vi "Initialize Daemon.vi"(8 "error in (no error)":errorcluster, 9 "data model":refnum<class "Device Data Model.lvclass">, 10 "transmission data unit":refnum<class "Transmission Data Unit.lvclass">, 11 "serial slave in":refnum<class "Serial Slave.lvclass">) -> (0 "error out":errorcluster, 3 "serial slave out":refnum<class "Serial Slave.lvclass">)   [LabVIEW 2018, in "SubVIs.lvlib" / "Serial Slave.lvclass"]
doc: "This provides an interface for the slave to launch a protocol daemon."
uses:
  Serial Slave.lvclass
  Transmission Data Unit.lvclass
  Device Data Model.lvclass
  Serial Data Unit.lvclass
  C:/OCC/ICM/Source Distributions/Buses/Transmission Data Unit.lvclass
  Serial Slave.lvclass/Serial Slave.ctl
  Transmission Data Unit.lvclass/Transmission Data Unit.ctl
  Read VISA resource name.vi
  Read Baud Rate.vi
  Read Parity.vi
  Read Flow Control.vi
  Network Slave.lvclass
  SubVIs.lvlib
  Serial Shared Components.lvlib
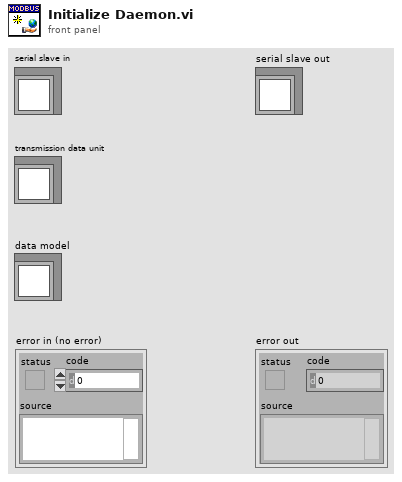
[diagram p1: front panel]
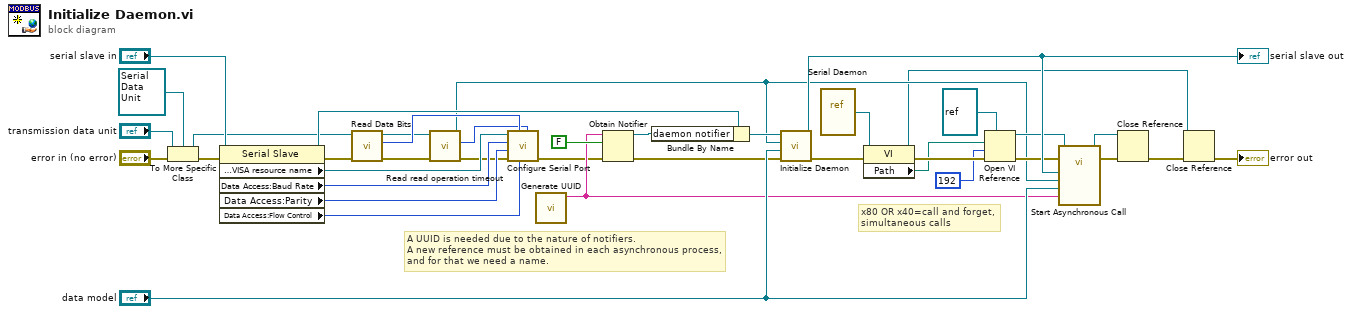
[diagram p0: block diagram]
diagram:
  # "x80 OR x40=call and forget,\nsimultaneous calls"
  # "A UUID is needed due to the nature of notifiers.\nA new reference must be obtained in each asynchronous process,\nand for that we need a name."
  n1 = To More Specific Class(target class=refnum<class "Serial Data Unit.lvclass"> refnum ("Serial Data Unit in"), reference="transmission data unit", error in="error in (no error)") -> (specific class reference=w21:refnum<class "Serial Data Unit.lvclass">, error out=w23:errorcluster)
  n2 = property class="Serial Slave"(reference="serial slave in", error in=w23) -> (reference out=w24:refnum<class "Serial Slave.lvclass">, error out=w33:errorcluster, "Data Access:VISA resource name"=w19:refnum<visa-resource-name>, "Data Access:Baud Rate"=w17:u32, "Data Access:Parity"=w16:u16, "Data Access:Flow Control"=w15:u16)
  n3 = call-dynamic "Read Data Bits.vi"("error in (no error)"=w33, "serial data unit in"=w21) -> ("error out"=w20:errorcluster, "data bits"=w18:u16, "serial data unit out"=w7:refnum<class "Serial Data Unit.lvclass">)  [unwired: 7 in]
  n4 = call "Read read operation timeout.vi"("error in (no error)"=w20, "transmission data unit in"=w7) -> ("error out"=w8:errorcluster, "read operation timeout"=w5:i32, "transmission data unit out"=w6:refnum<class "Serial Data Unit.lvclass">)  [unwired: 7 in]
  n5 = call "Configure Serial Port.vi"("Timeout"=w5, "flow control"=w15, "data bits"=w18, "error in (no error)"=w8, "parity"=w16, "baud rate"=w17, "VISA refnum in"=w19) -> ("error out"=w14:errorcluster)  [unwired: 4 in]
  n6 = call "Generate UUID.vi"() -> ("UUID"=w25:string)  [unwired: 11 in]
  n7 = Obtain Notifier(name (unnamed)=w25, notification data type=FALSE, error in (no error)=w14) -> (notifier out=w26:refnum<notifier>, error out=w11:errorcluster)  [unwired: 1 in, 1 out]
  n8 = Bundle By Name(cluster=w24, "daemon notifier"=w26) -> (w9:refnum<class "Serial Slave.lvclass">)
  n9 = call-parent "Initialize Daemon.vi"("error in (no error)"=w11, "data model"="data model", "transmission data unit"=w6, "network slave in"=w9) -> ("error out"=w10:errorcluster, "network slave out"=w36:refnum<class "Serial Slave.lvclass">)  [unwired: 6 in]
  "serial slave out" <- w36
  n10 = vi-ref "Serial Daemon.vi"() -> (w32:refnum<vi>)
  n11 = property class="VI"(reference=w32, error in=w10) -> (reference out=w1:refnum<vi>, error out=w31:errorcluster, "Path"=w30:path)
  n12 = Open VI Reference(type specifier VI Refnum (for type only)=refnum<vi> refnum, vi path=w30, options=192 ("x .or. y?"), error in (no error)=w31) -> (vi reference=w29:refnum<vi>, error out=w27:errorcluster)  [unwired: 2 in]
  n13 = call-by-ref "Start Asynchronous Call"(reference=w29, error in=w27, "UUID"=w25, "Data Model"="data model", "transmission data unit"=w6, "serial slave"=w36) -> (reference out=w3:refnum<vi>, error out=w37:errorcluster)  [unwired: 8 in]
  n14 = Close Reference(reference=w3, error in (no error)=w37) -> (error out=w4:errorcluster)
  n15 = Close Reference(reference=w1, error in (no error)=w4) -> (error out=→"error out":errorcluster)
